vi "Teleop.vi"(10 "Match Info":T2={"Autonomous Elapsed Seconds"=0.0, "TeleOp Elapsed Seconds"=0.0, "Disabled Elapsed Seconds"=0.0, "Visited Autonomous"=FALSE, "Visited TeleOp"=FALSE, "Visited Disabled"=FALSE, "Autonomous Settings"={"Autonomous Style"=enum."Independent", "VI Refnum"=refnum}}, 11 "Call Context":T3) -> ()   [LabVIEW 2020]
doc: "This VI is called for each TeleOp packet received from the DS where the robot is not disabled. It is often used to read from the joysticks and update I/O or to update setpoints for timed control loops. It should complete and return within 20 milliseconds or it may miss DS packets."
uses:
  <vilib>/Rock Robotics/WPI/DriverStation/WPI_DriverStationDerivedRobotMode.ctl
  <vilib>/Rock Robotics/WPI/DriverStation/WPI_DriverStationMatch Info.ctl
  <vilib>/Rock Robotics/WPI/ThirdParty/Phoenix-LabVIEW/Motor Controller/Controls/CTRE_Phoenix_MotorControl_ControlMode.ctl
  <vilib>/Rock Robotics/WPI/Solenoid/WPI_SolenoidValue.ctl
  <vilib>/Rock Robotics/WPI/Utilities/WPI_GetSetVariantRefNum.vi
  <vilib>/Rock Robotics/Network Tables/NT Read Boolean.vi
  <vilib>/Rock Robotics/Network Tables/NT Read Number.vi
  <vilib>/Rock Robotics/WPI/Solenoid/WPI_SolenoidSetEnum.vi
  <vilib>/Rock Robotics/WPI/ThirdParty/Phoenix-LabVIEW/Motor Controller/Get/CTRE_Phoenix_MotorController_IntegratedSensorData_TalonFX.vi
  <vilib>/addons/control/pid/pid.llb/PID (DBL).vi
  <vilib>/Rock Robotics/Network Tables/NT Write Number.vi
  <vilib>/addons/control/pid/NI_PID_pid.lvlib
panel:
  in  "PID gains 5":T1={"proportional gain (Kc)"=0.005, "integral time (Ti, min)"=0.0, "derivative time (Td, min)"=2e-05} {"derivative time (Td, min)" format="%.6f"; "integral time (Ti, min)" format="%.3f"; "proportional gain (Kc)" format="%.3f"}
  in  "Subtract rpm":dbl=2975.0
  out "% voltage":dbl
  out "voltage (V)":dbl
  out "Motor Volts":dbl
  out "rpm":dbl
  out "limelight tx":dbl
  out "limelight ty":dbl
  in  "Auto-Accept":bool
  in  "8togglePressed?":bool
  out "Sample Slider 0":dbl(slide) scale=0.0..5.0
  out "Sample Boolean 1":bool
  out "Sample Boolean 0":bool
  # "-1"
  # "0"
  # ".75"
  # ".75"
  # "-.6"
  # "-.35"
  # ".1"
  # "1"
  # "-.1"
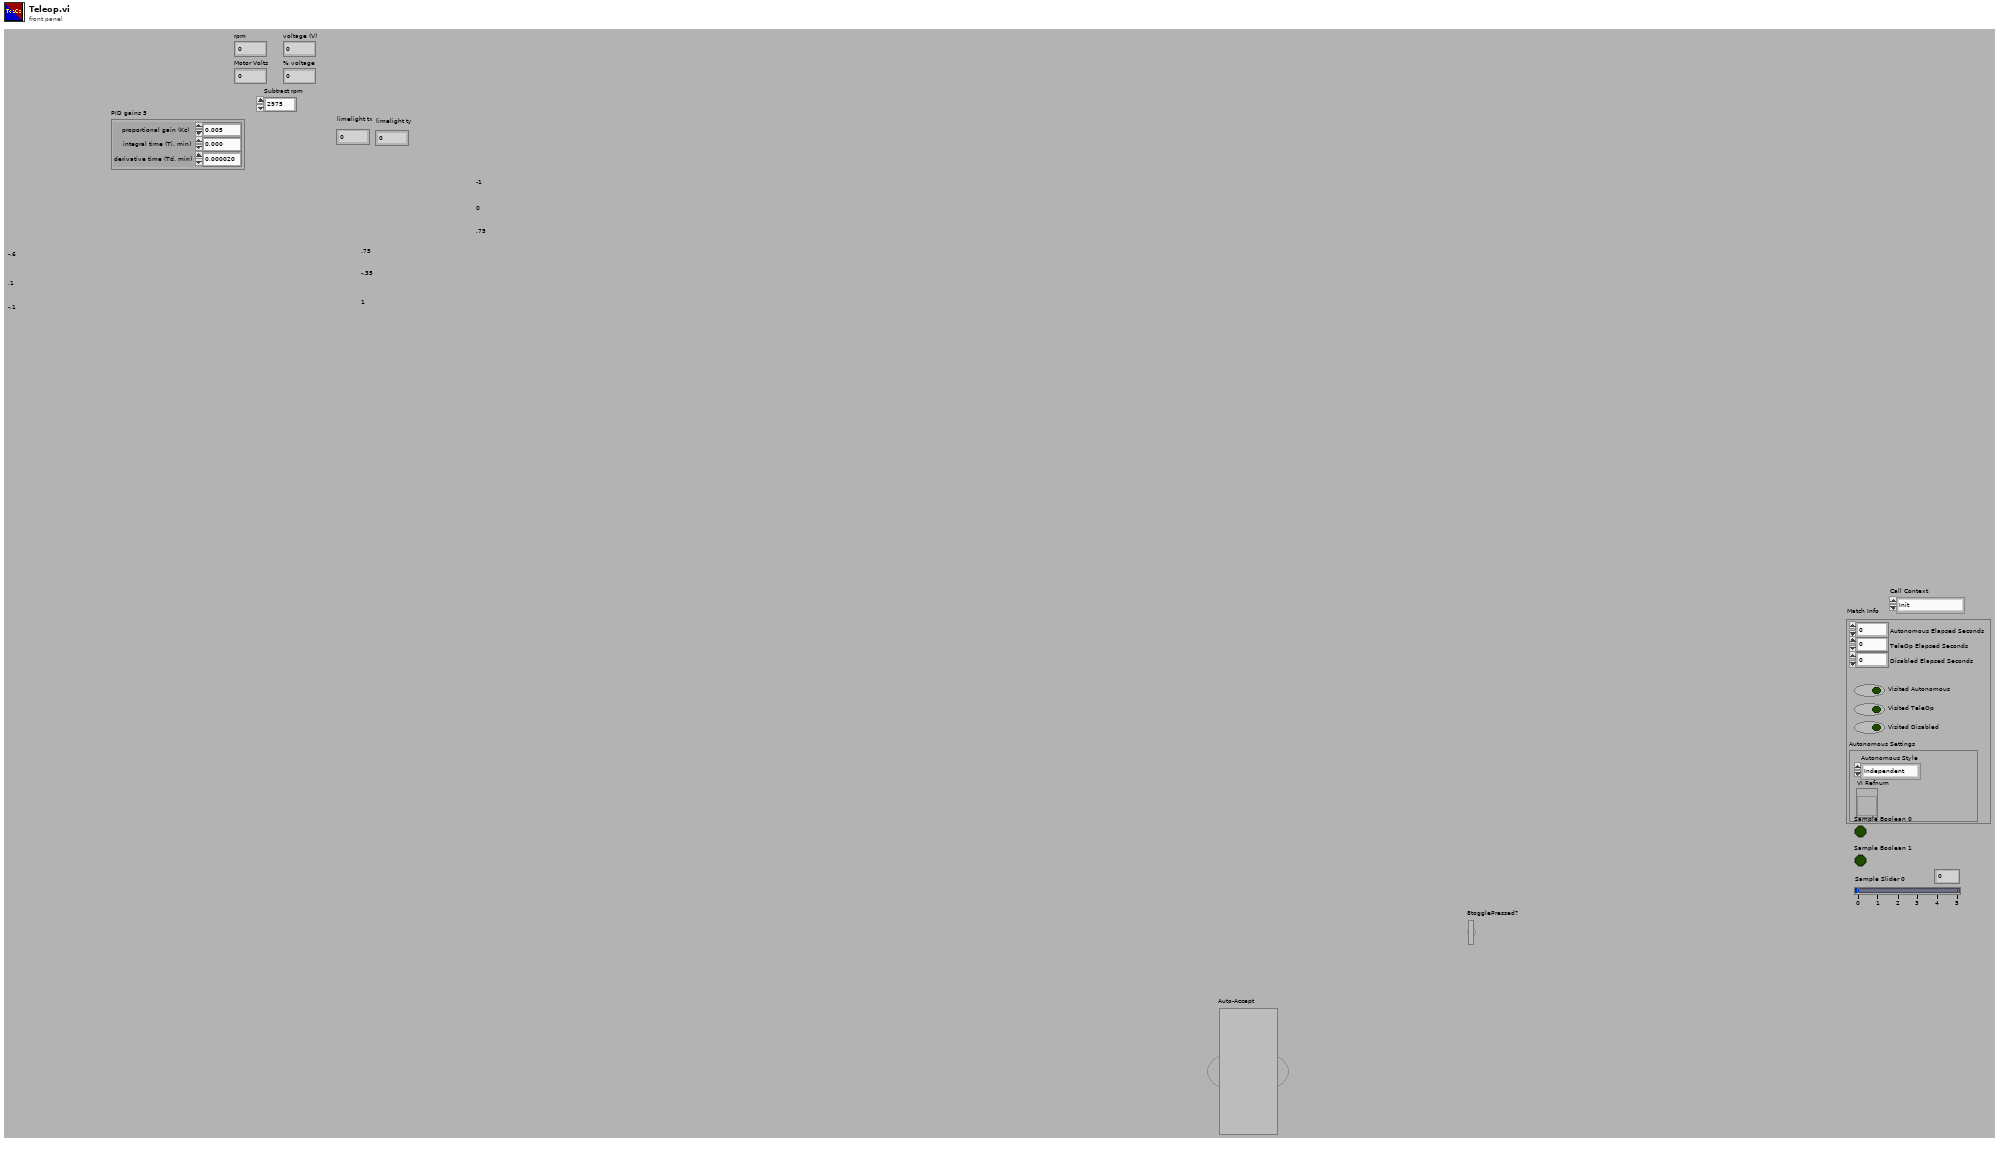
[diagram p1: front panel]
types:
  T1 = cluster{"proportional gain (Kc)":dbl, "integral time (Ti, min)":dbl, "derivative time (Td, min)":dbl}
  T2 = typedef "WPI_DriverStationMatch Info.ctl" = cluster{"Autonomous Elapsed Seconds":dbl, "TeleOp Elapsed Seconds":dbl, "Disabled Elapsed Seconds":dbl, "Visited Autonomous":bool, "Visited TeleOp":bool, "Visited Disabled":bool, "Autonomous Settings":cluster{"Autonomous Style":enum16{"Iterative", "Independent"}, "VI Refnum":refnum<vi>}}
  T3 = typedef "WPI_DriverStationDerivedRobotMode.ctl" = enum16{"Init", "Execute", "Stop"}
  T4 = typedef "CTRE_Phoenix_MotorControl_ControlMode.ctl" = u16
  T5 = typedef "WPI_SolenoidValue.ctl" = enum16{"Off", "On", "Forward", "Reverse"}
  T6 = typedef "WPI_MotorControlDeviceRef.ctl" = cluster{"DeviceStatus":errorcluster, "Type":T7, "PWM":cluster{"PWM Channel":T8, "DeadBand":T9}, "CAN":cluster{"Device Number":u8, "SetOutput VI Ref":variant, "GetOutput VI Ref":variant, "Enable VI Ref":variant, "Disable VI Ref":variant, "Data":variant}, "Invert":bool, "DIO PWM":cluster{"PWM \"Enable\" Channel":T8, "DIOChannel":T10, "PWM Rate":dbl}}
  T7 = typedef "WPI_MotorControlType.ctl" = enum16{"PWM", "CAN", "DIO PWM"}
  T8 = typedef "FPGA_DIOPWMChannel.ctl" = enum8{"PWM 0", "PWM 1", "PWM 2", "PWM 3", "PWM 4", "PWM 5", "PWM 6", "PWM 7", "PWM 8", "PWM 9", "PWM MXP 0", "PWM MXP 1", "PWM MXP 2", "PWM MXP 3", "PWM MXP 4", "PWM MXP 5", "PWM MXP 6", "PWM MXP 7", "PWM MXP 8", "PWM MXP 9", "Invalid"}
  T9 = typedef "WPI_PWMDeadband.ctl" = cluster{"Name":string, "maxPositivePwm":i32, "minPositivePwm":i32, "centerPwm":i32, "maxNegativePwm":i32, "minNegativePwm":i32, "angularRange":u16}
  T10 = typedef "FPGA_DIOChannel.ctl" = enum8{"DIO 0", "DIO 1", "DIO 2", "DIO 3", "DIO 4", "DIO 5", "DIO 6", "DIO 7", "DIO 8", "DIO 9", "DIO MXP 0", "DIO MXP 1", "DIO MXP 2", "DIO MXP 3", "DIO MXP 4", "DIO MXP 5", "DIO MXP 6", "DIO MXP 7", "DIO MXP 8", "DIO MXP 9", "DIO MXP 10", "DIO MXP 11", "DIO MXP 12", "DIO MXP 13", "DIO MXP 14", "DIO MXP 15", "SPI Port CS1", "SPI Port CS2", "SPI Port CS3", "SPI Port MISO", "SPI Port MOSI", "Invalid"}
  T11 = typedef "WPI_SolenoidDevRef.ctl" = cluster{"DevStatus":errorcluster, "Pneumatics Control Module":u8, "Forward Solenoid Channel":T12, "Reverse Solenoid Channel":T12}
  T12 = typedef "WPI_SolenoidChannel.ctl" = enum8{"Solenoid 0", "Solenoid 1", "Solenoid 2", "Solenoid 3", "Solenoid 4", "Solenoid 5", "Solenoid 6", "Solenoid 7", "Solenoid 8", "Solenoid 9", "Solenoid 10", "Solenoid 11", "Solenoid 12", "Solenoid 13", "Solenoid 14", "Solenoid 15", "Invalid"}
  T13 = typedef "WPI_CompressorDevRef.ctl" = cluster{"DevStatus":errorcluster, "Pneumatics Control Module":u8}
  T14 = typedef "WPI_SwitchDevRef.ctl" = cluster{"DevStatus":errorcluster, "DIO Channel":T10, "CntIndex":T15, "Normally Closed":bool}
  T15 = typedef "FPGA_CounterCtrSystemIndex.ctl" = enum8{"Ctr 0", "Ctr 1", "Ctr 2", "Ctr 3", "Ctr 4", "Ctr 5", "Ctr 6", "Ctr 7", "Invalid"}
  T16 = typedef "WPI_JoystickDevRef.ctl" = cluster{"Device":T17}
  T17 = typedef "WPI_JoystickDeviceEnum.ctl" = enum16{"USB 0", "USB 1", "USB 2", "USB 3", "USB 4", "USB 5"}
  T18 = cluster{"A":bool, "B":bool, "X":bool, "Y":bool, "Left Bumper":bool, "Right Bumper":bool, "View Button":bool, "Menu Button":bool, "Left Joystick Press":bool, "Right Joystick Press":bool, "Left Thumbpad X Axis":dbl, "Left Thumbpad Y Axis":dbl, "Left Trigger":dbl, "Right Trigger":dbl, "Right Thumbpad X Axis":dbl, "Right Thumbpad Y Axis":dbl, "Driver - Trigger":bool, "Driver - Middle Thumb":bool, "Driver - Left Thumb":bool, "Driver - Right Thumb":bool, "Driver - Left Top Left ":bool, "Driver - Left Top Middle":bool, "Driver - Left Top Right":bool, "Driver - Left Bottom Right":bool, "Driver - Left Bottom Middle":bool, "Driver - Left Bottom Left":bool, "Driver - Right Top Right":bool, "Driver - Right Top Middle":bool, "Driver - Right Top Left":bool, "Driver - Right Bottom Left":bool, "Driver - Right Bottom Middle":bool, "Driver - Right Bottom Right":bool, "Driver - X Axis":dbl, "Driver - Y Axis":dbl, "Driver - Z Axis":dbl}
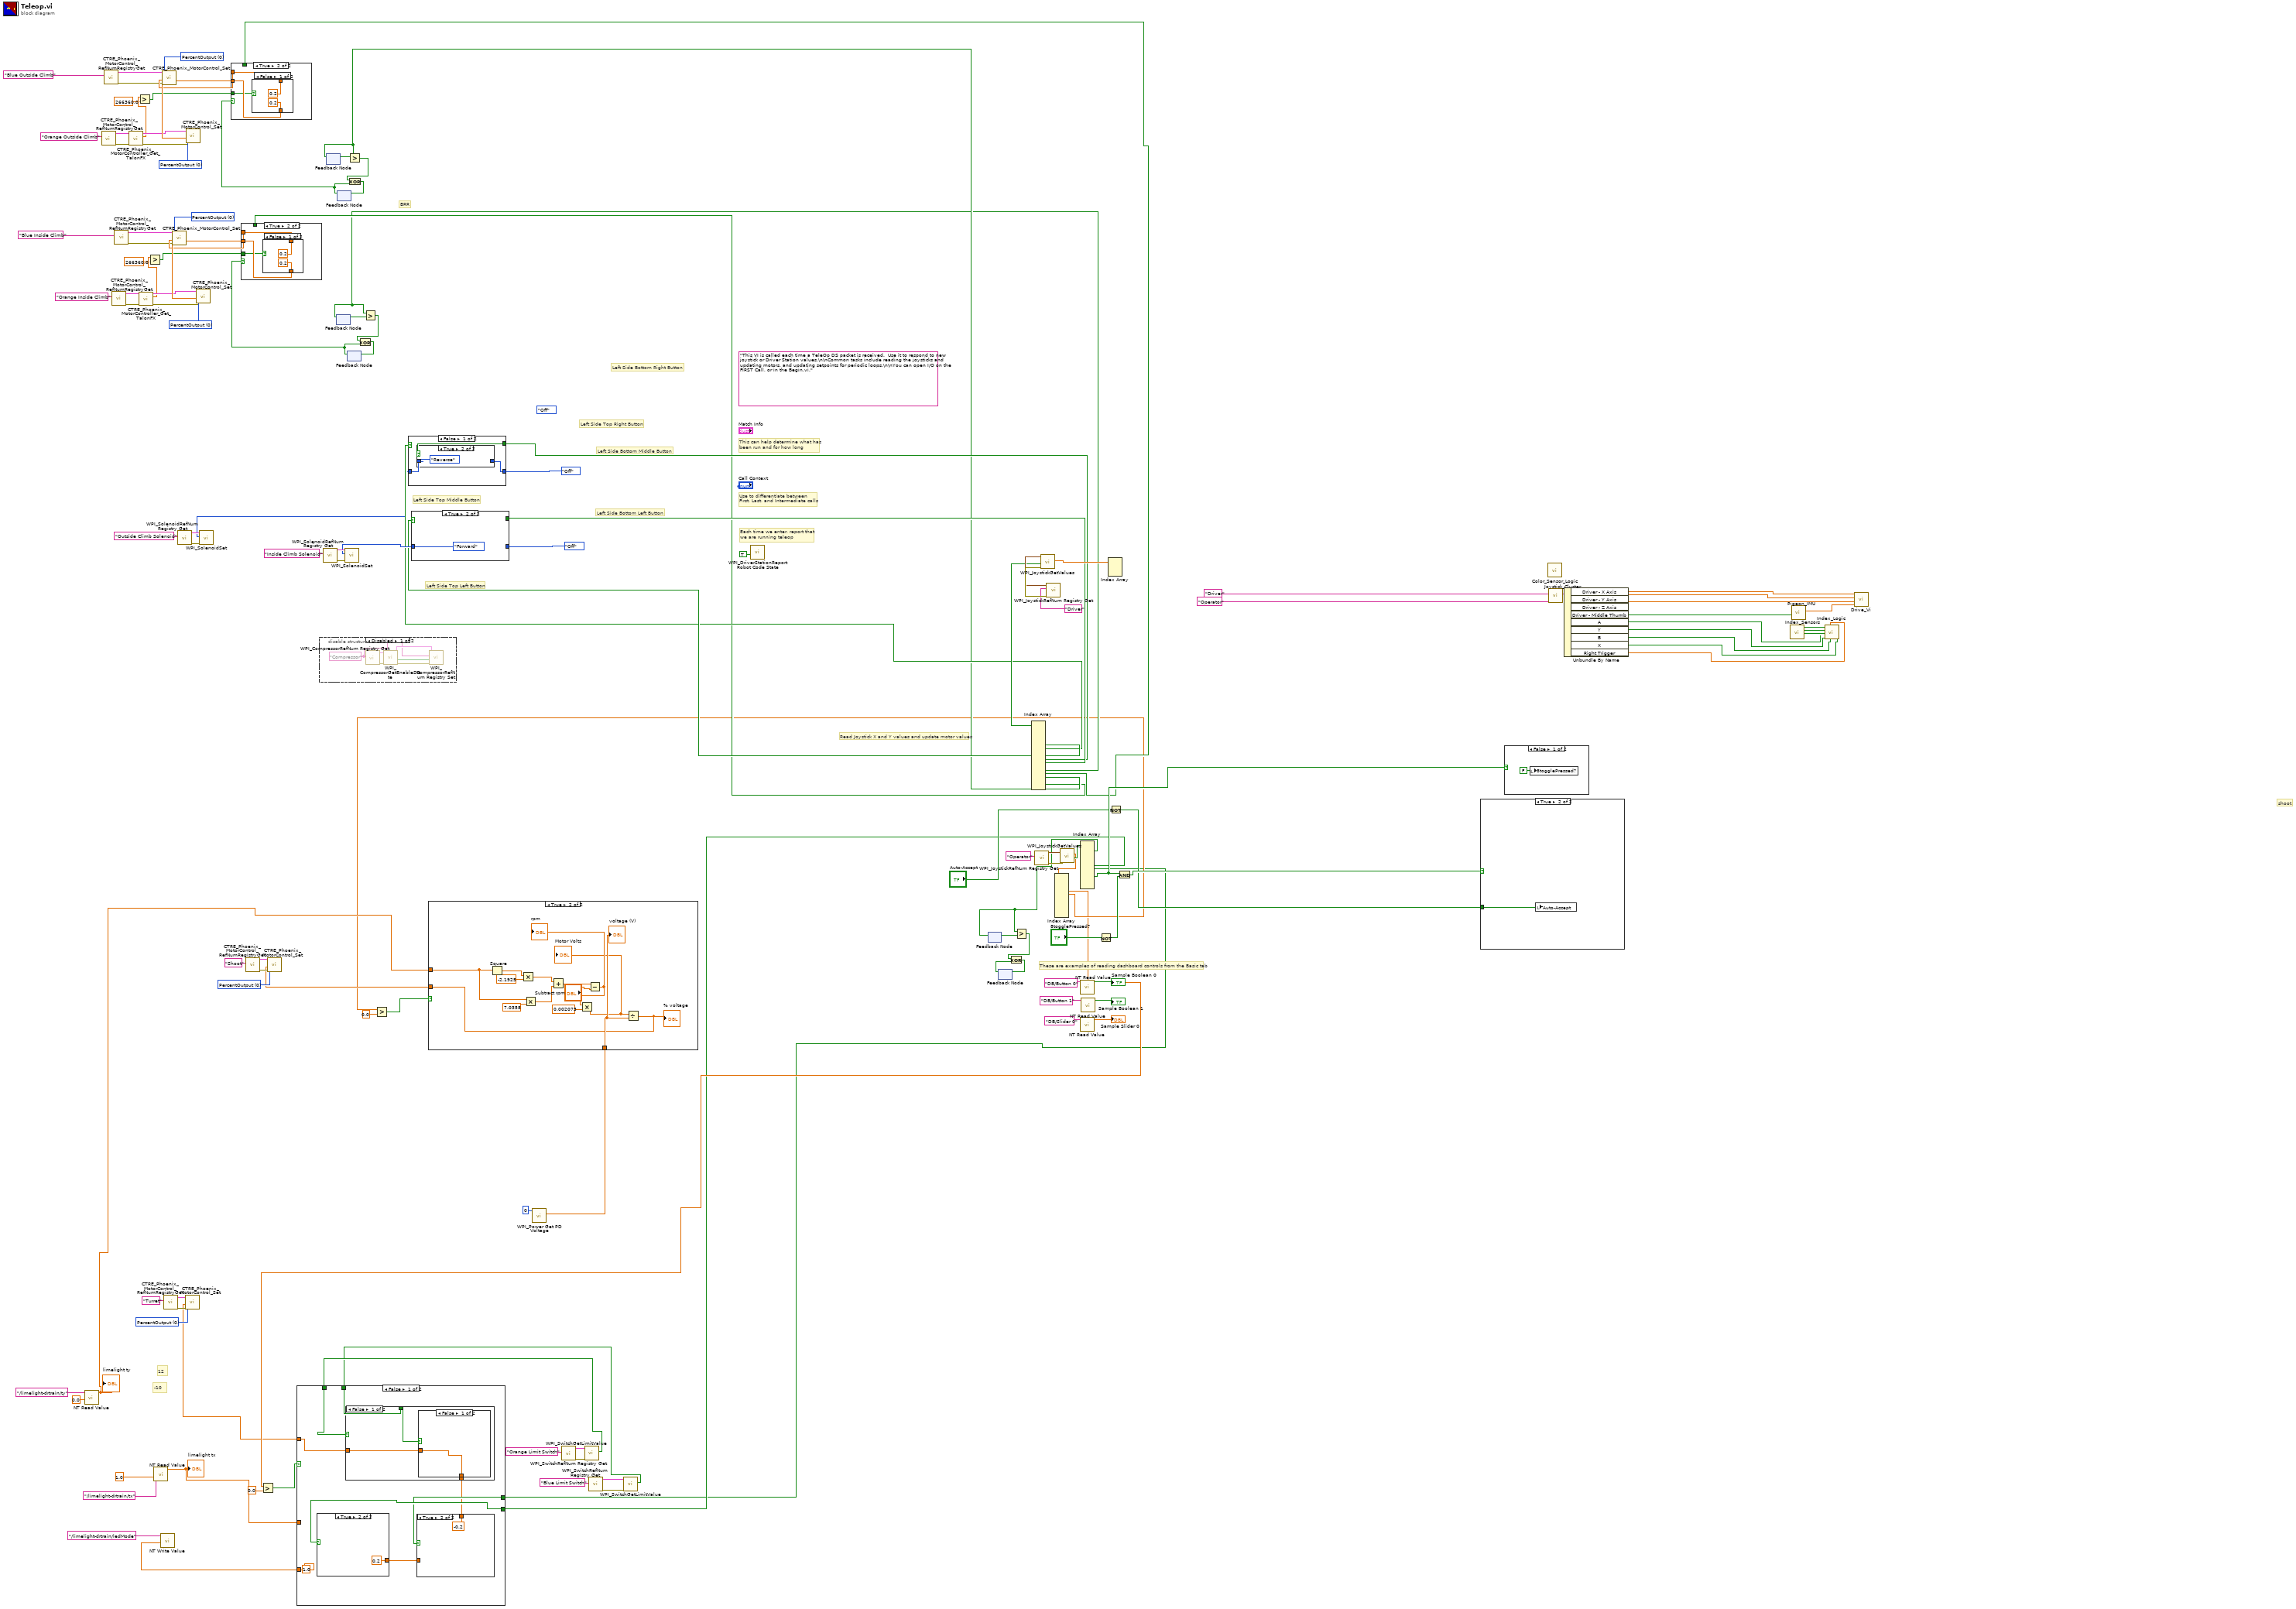
[diagram p0: block diagram]
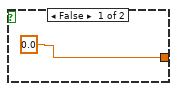
[diagram p3: hidden frame]
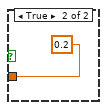
[diagram p4: hidden frame]
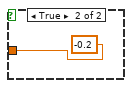
[diagram p5: hidden frame]
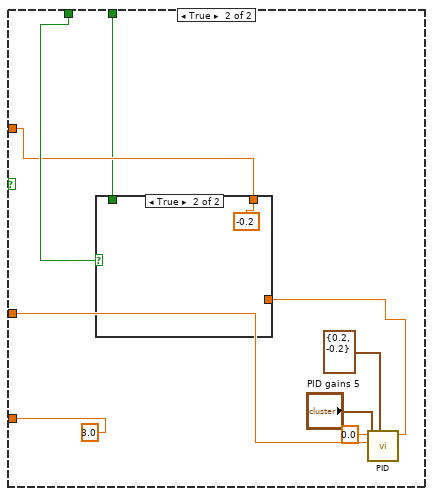
[diagram p6: hidden frame]
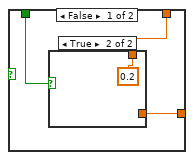
[diagram p7: hidden frame]
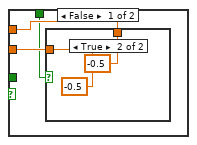
[diagram p9: hidden frame]
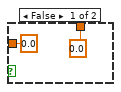
[diagram p10: hidden frame]
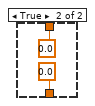
[diagram p11: hidden frame]
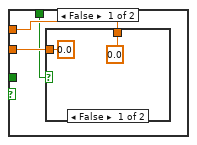
[diagram p12: hidden frame]
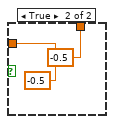
[diagram p13: hidden frame]
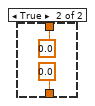
[diagram p14: hidden frame]
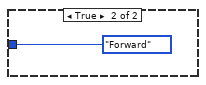
[diagram p17: hidden frame]
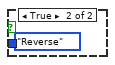
[diagram p19: hidden frame]
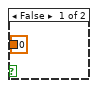
[diagram p20: hidden frame]
diagram:
  w52 = T4 0 items=["PercentOutput"=0, "Position"=1, "Velocity"=2, "Current"=3, "Follower"=5, "MotionProfile"=6, "MotionMagic"=7, "MotionProfileArc"=10, "Disabled"=15] ("Control Mode")
  w53 = T4 0 items=["PercentOutput"=0, "Position"=1, "Velocity"=2, "Current"=3, "Follower"=5, "MotionProfile"=6, "MotionMagic"=7, "MotionProfileArc"=10, "Disabled"=15] ("Control Mode")
  (unwired) WPI_SolenoidValue."Off" ("inside climb start")
  w71 = T4 0 items=["PercentOutput"=0, "Position"=1, "Velocity"=2, "Current"=3, "Follower"=5, "MotionProfile"=6, "MotionMagic"=7, "MotionProfileArc"=10, "Disabled"=15] ("Control Mode")
  w72 = T4 0 items=["PercentOutput"=0, "Position"=1, "Velocity"=2, "Current"=3, "Follower"=5, "MotionProfile"=6, "MotionMagic"=7, "MotionProfileArc"=10, "Disabled"=15] ("Control Mode")
  w102 = T4 0 items=["PercentOutput"=0, "Position"=1, "Velocity"=2, "Current"=3, "Follower"=5, "MotionProfile"=6, "MotionMagic"=7, "MotionProfileArc"=10, "Disabled"=15] ("Control Mode")
  w107 = T4 0 items=["PercentOutput"=0, "Position"=1, "Velocity"=2, "Current"=3, "Follower"=5, "MotionProfile"=6, "MotionMagic"=7, "MotionProfileArc"=10, "Disabled"=15] ("Control Mode")
  (unwired) "This VI is called each time a TeleOp DS packet is received.  Use it to respond to new joystick or Driver Station values.\n\nCommon tasks include reading the joysticks and updating motors, and updating setpoints for periodic loops.\n\nYou can open I/O on the FIRST Call, or in the Begin.vi."
  # "BRR"
  # "Left Side Bottom Right Button"
  # "Left Side Top Right Button"
  # "Left Side Bottom Middle Button"
  # "Left Side Top Middle Button"
  # "Left Side Bottom Left Button"
  # "Left Side Top Left Button"
  # "shoot"
  # "12"
  # "-10"
  # "These are examples of reading dashboard controls from the Basic tab"
  # "Read Joystick X and Y values and update motor values"
  # "Each time we enter, report that\nwe are running teleop"
  # "Use to differentiate between\nFirst, Last, and Intermediate calls"
  # "This can help determine what has\nbeen run and for how long"
  n1 = call-poly <vilib>:"NT Read Value.vi"("Default Value"=0.0, "Name"="/limelight-drtrain/ty") -> ("Numeric"=w83:dbl)  [unwired: 8 in, 1 out]
  "limelight ty" <- w83
  n2 = call <vilib>:"CTRE_Phoenix_MotorControl_RefNumRegistryGet.vi"("refnum name"="Orange Outside Climb") -> ("error out"=w49:errorcluster, "PhoenixMotorControlDevRef"=w48:T6)  [unwired: 9 in]
  n3 = call <vilib>:"CTRE_Phoenix_MotorControl_RefNumRegistryGet.vi"("refnum name"="Blue Outside Climb") -> ("error out"=w44:errorcluster, "PhoenixMotorControlDevRef"=w45:T6)  [unwired: 9 in]
  n4 = call <vilib>:"CTRE_Phoenix_MotorControl_RefNumRegistryGet.vi"("refnum name"="Orange Inside Climb") -> ("error out"=w68:errorcluster, "PhoenixMotorControlDevRef"=w67:T6)  [unwired: 9 in]
  n5 = call <vilib>:"CTRE_Phoenix_MotorControl_RefNumRegistryGet.vi"("refnum name"="Blue Inside Climb") -> ("error out"=w63:errorcluster, "PhoenixMotorControlDevRef"=w64:T6)  [unwired: 9 in]
  n6 = call-poly <vilib>:"CTRE_Phoenix_MotorController_Get_TalonFX.vi"("PhoenixMotorControlDevRef"=w48, "error in"=w49) -> ("PhoenixMotorControlDevRef"=w47:T6, "Position"=w39:dbl, "error out"=w46:errorcluster)  [unwired: 9 in, 2 out]
  n7 = Greater?(x=w39, y=266360.0) -> (0:w37:bool)
  n8 = call-poly <vilib>:"CTRE_Phoenix_MotorController_Get_TalonFX.vi"("PhoenixMotorControlDevRef"=w67, "error in"=w68) -> ("PhoenixMotorControlDevRef"=w66:T6, "Position"=w58:dbl, "error out"=w65:errorcluster)  [unwired: 9 in, 2 out]
  n9 = Greater?(x=w58, y=266360.0) -> (0:w56:bool)
  n10 = call-poly <vilib>:"NT Read Value.vi"("Default Value"=1.0, "Name"="/limelight-drtrain/tx") -> ("Numeric"=w24:dbl)  [unwired: 8 in, 1 out]
  "limelight tx" <- w24
  n11 = call <vilib>:"CTRE_Phoenix_MotorControl_RefNumRegistryGet.vi"("refnum name"="Turret") -> ("error out"=w105:errorcluster, "PhoenixMotorControlDevRef"=w104:T6)  [unwired: 9 in]
  n12 = call <vilib>:"WPI_SolenoidRefNum Registry Get.vi"("refnum name"="Outside Climb Solenoid") -> ("error out"=w97:errorcluster, "SolenoidDevRef"=w96:T11)  [unwired: 9 in]
  n13 = call <vilib>:"CTRE_Phoenix_MotorControl_RefNumRegistryGet.vi"("refnum name"="Shoot") -> ("error out"=w110:errorcluster, "PhoenixMotorControlDevRef"=w109:T6)  [unwired: 9 in]
  n14 = disable-structure shown="Disabled" {
    frame Disabled {
      w137 = "Compressor" ("refnum name")
      n15 = call <vilib>:"WPI_CompressorRefNum Registry Get.vi"("refnum name"=w137) -> ("error out"=w142:errorcluster, "CompressorDevRef"=w141:T13)  [unwired: 9 in]
      n16 = call <vilib>:"WPI_CompressorGetEnableState.vi"("error in (no error)"=w142, "CompressorDevRef"=w141) -> ("error out"=w140:errorcluster, "Compressor Running"=w139:bool, "CompressorDevRef"=w138:T13)  [unwired: 3 in, 4 out]
      n17 = call <vilib>:"WPI_CompressorRefNum Registry Set.vi"("error in (no error)"=w140, "Test Mode Only"=w139, "refnum name"=w137, "CompressorDevRef"=w138) -> ()  [unwired: 6 in, 2 out]
    }
    frame Enabled {
    }
  }
  n18 = call <vilib>:"WPI_SolenoidRefNum Registry Get.vi"("refnum name"="Inside Climb Solenoid") -> ("error out"=w94:errorcluster, "SolenoidDevRef"=w93:T11)  [unwired: 9 in]
  n19 = feedback #1() -> (w43:bool)  [unwired: 1 in]
  n20 = feedback #2() -> (w62:bool)  [unwired: 1 in]
  n21 = feedback #3() -> (w40:bool)  [unwired: 1 in]
  n22 = feedback #4() -> (w59:bool)  [unwired: 1 in]
  n23 = call <vilib>:"WPI_Power Get PD Voltage.vi"("Power Distribution Panel (def)"=u8 0) -> ("voltage (V)"=w84:dbl)  [unwired: 13 in, 1 out]
  n24 = call <vilib>:"WPI_SwitchRefNum Registry Get.vi"("refnum name"="Orange Limit Switch") -> ("error out"=w91:errorcluster, "SwitchDevRef"=w90:T14)  [unwired: 9 in]
  n25 = call <vilib>:"WPI_SwitchGetLimitValue.vi"("error in (no error)"=w91, "SwitchDevRef"=w90) -> ("Switch Pressed"=w22:bool)  [unwired: 7 in, 2 out]
  n26 = call <vilib>:"WPI_SwitchRefNum Registry Get.vi"("refnum name"="Blue Limit Switch") -> ("error out"=w88:errorcluster, "SwitchDevRef"=w87:T14)  [unwired: 9 in]
  n27 = call <vilib>:"WPI_SwitchGetLimitValue.vi"("error in (no error)"=w88, "SwitchDevRef"=w87) -> ("Switch Pressed"=w21:bool)  [unwired: 7 in, 2 out]
  n28 = call <vilib>:"WPI_DriverStationReport Robot Code State.vi"("TeleOp"=TRUE ("Autonomous")) -> ()  [unwired: 10 in, 1 out]
  n29 = feedback #5() -> (w114:bool)  [unwired: 1 in]
  n30 = feedback #6() -> (w36:bool)  [unwired: 1 in]
  n31 = call <vilib>:"WPI_JoystickRefNum Registry Get.vi"("refnum name"="Operator") -> ("error out"=w123:errorcluster, "JoystickDevRef"=w122:T16)  [unwired: 9 in]
  n32 = call <vilib>:"WPI_JoystickRefNum Registry Get.vi"("refnum name"="Driver") -> ("error out"=w135:errorcluster, "JoystickDevRef"=w134:T16)  [unwired: 9 in]
  n33 = call <vilib>:"WPI_JoystickGetValues.vi"("error in (no error)"=w135, "JoystickDevRef"=w134) -> ("Buttons"=w131:bool[], "Axes"=w132:dbl[])  [unwired: 5 in, 3 out]
  n34 = Index Array(array=w131) -> (element #5=w79:bool, element #6=w77:bool, element #9=w76:bool, element #10=w80:bool, element #12=w32:bool, element #13=w35:bool, element #14=w34:bool, element #16=w33:bool)  [unwired: 17 in, 9 out]
  n35 = case shown="True" w40 {
    tunnel: [w144 w151] -> w51
    tunnel: [w145 w152] -> w50
    tunnel: w35 -> [w143 _]
    tunnel: w37 -> [_ w150]
    frame False {
      n36 = case shown="True" w143 {
        tunnel: [0.0 ("Output") -0.5 ("Output")] -> w145
        tunnel: [0.0 ("Output") -0.5 ("Output")] -> w144
        frame False {
        }
        frame True {
        }
      }
    }
    frame True {
      n37 = case shown="False" w150 {
        tunnel: [0.2 ("Output") 0.0 ("Output")] -> w152
        tunnel: [0.2 ("Output") 0.0 ("Output")] -> w151
        frame False {
        }
        frame True {
        }
      }
    }
  }
  n38 = call <vilib>:"CTRE_Phoenix_MotorControl_Set.vi"("error in (no error)"=w44, "Output"=w50, "Control Mode"=w53, "PhoenixMotorControlDevRef"=w45) -> ()  [unwired: 6 in, 2 out]
  n39 = call <vilib>:"CTRE_Phoenix_MotorControl_Set.vi"("error in (no error)"=w46, "Output"=w51, "Control Mode"=w52, "PhoenixMotorControlDevRef"=w47) -> ()  [unwired: 6 in, 2 out]
  n40 = case shown="True" w59 {
    tunnel: [w158 w165] -> w70
    tunnel: [w159 w166] -> w69
    tunnel: w33 -> [w157 _]
    tunnel: w56 -> [_ w164]
    frame False {
      n41 = case shown="False" w157 {
        tunnel: [0.0 ("Output") -0.5 ("Output")] -> w159
        tunnel: [0.0 ("Output") -0.5 ("Output")] -> w158
        frame False {
        }
        frame True {
        }
      }
    }
    frame True {
      n42 = case shown="False" w164 {
        tunnel: [0.2 ("Output") 0.0 ("Output")] -> w166
        tunnel: [0.2 ("Output") 0.0 ("Output")] -> w165
        frame False {
        }
        frame True {
        }
      }
    }
  }
  n43 = call <vilib>:"CTRE_Phoenix_MotorControl_Set.vi"("error in (no error)"=w63, "Output"=w69, "Control Mode"=w72, "PhoenixMotorControlDevRef"=w64) -> ()  [unwired: 6 in, 2 out]
  n44 = call <vilib>:"CTRE_Phoenix_MotorControl_Set.vi"("error in (no error)"=w65, "Output"=w70, "Control Mode"=w71, "PhoenixMotorControlDevRef"=w66) -> ()  [unwired: 6 in, 2 out]
  n45 = feedback-in #1(w34) -> ()
  n46 = feedback-in #2(w32) -> ()
  n47 = Greater?(x=w34, y=w43) -> (0:w42:bool)
  n48 = Exclusive Or(1:w40, 2:w42) -> (0:w41:bool)
  n49 = feedback-in #3(w41) -> ()
  n50 = Greater?(x=w32, y=w62) -> (0:w61:bool)
  n51 = Exclusive Or(1:w59, 2:w61) -> (0:w60:bool)
  n52 = feedback-in #4(w60) -> ()
  n53 = case shown="False" w77 {
    tunnel: [w171 WPI_SolenoidValue."Forward" ("inside climb start")] -> w75
    tunnel: WPI_SolenoidValue."Off" ("inside climb start") -> [w172 _]
    tunnel: w76 -> [w173 _]
    frame False {
      n54 = case shown="True" w173 {
        tunnel: w172 -> [w174 _]
        tunnel: [w174 WPI_SolenoidValue."Reverse" ("inside climb start")] -> w171
        frame False {
        }
        frame True {
        }
      }
    }
    frame True {
    }
  }
  n55 = call-poly <vilib>:"WPI_SolenoidSet.vi"("error in (no error)"=w97, "Value"=w75, "SolenoidDevRef"=w96) -> ()  [unwired: 7 in, 2 out]
  n56 = case shown="True" w79 {
    tunnel: [w177 WPI_SolenoidValue."Forward" ("inside climb start")] -> w82
    tunnel: WPI_SolenoidValue."Off" ("inside climb start") -> [w178 _]
    tunnel: w80 -> [w179 _]
    frame False {
      n57 = case shown="False" w179 {
        tunnel: w178 -> [w180 _]
        tunnel: [w180 WPI_SolenoidValue."Reverse" ("inside climb start")] -> w177
        frame False {
        }
        frame True {
        }
      }
    }
    frame True {
    }
  }
  n58 = call-poly <vilib>:"WPI_SolenoidSet.vi"("error in (no error)"=w94, "Value"=w82, "SolenoidDevRef"=w93) -> ()  [unwired: 7 in, 2 out]
  n59 = call <vilib>:"WPI_JoystickGetValues.vi"("error in (no error)"=w123, "JoystickDevRef"=w122) -> ("Buttons"=w121:bool[], "Axes"=w31:dbl[])  [unwired: 5 in, 3 out]
  n60 = Index Array(array=w31) -> (element #3=w25:dbl, element #4=w28:dbl)  [unwired: 10 in, 8 out]
  n61 = Greater?(x=w25, y=0.0) -> (0:w26:bool)
  n62 = Greater?(x=w28, y=0.0) -> (0:w29:bool)
  n63 = case shown="True" w29 {
    tunnel: [0.0 ("Shoot %") w185] -> w106
    tunnel: w83 -> [_ w193]
    tunnel: w84 -> [_ w187]
    frame False {
    }
    frame True {
      n64 = Square(x=w193) -> (x^2=w196:dbl)
      n65 = Multiply(x=w196, y=-2.1925) -> (x*y=w194:dbl)
      n66 = Multiply(x=w193, y=7.0358) -> (x*y=w191:dbl)
      n67 = Add(x=w194, y=w191) -> (x+y=w190:dbl)
      n68 = Subtract(x=w190, y="Subtract rpm") -> (x-y=w189:dbl)
      "rpm" <- w189
      n69 = Multiply(x=w189, y=0.002075) -> (x*y=w186:dbl)
      "Motor Volts" <- w186
      n70 = Divide(x=w186, y=w187) -> (x/y=w185:dbl)
      "% voltage" <- w185
      "voltage (V)" <- w187
    }
  }
  n71 = call <vilib>:"CTRE_Phoenix_MotorControl_Set.vi"("error in (no error)"=w110, "Output"=w106, "Control Mode"=w107, "PhoenixMotorControlDevRef"=w109) -> ()  [unwired: 6 in, 2 out]
  n72 = Index Array(array=w121) -> (element #1=w113:bool, element #5=w20:bool, element #6=w19:bool, element #8=w116:bool)  [unwired: 11 in, 7 out]
  n73 = case shown="False" w26 {
    tunnel: w24 -> [_ w223]
    tunnel: [w198 w218] -> w23
    tunnel: w22 -> [w204 w219]
    tunnel: w21 -> [w203 w216]
    tunnel: w20 -> [w202 _]
    tunnel: w19 -> [w201 _]
    tunnel: [1.0 ("Numeric") 3.0 ("Numeric")] -> w17
    frame False {
      n74 = case shown="True" w202 {
        tunnel: [0.0 ("output") 0.2 ("output")] -> w200
        frame False {
        }
        frame True {
        }
      }
      n75 = case shown="True" w201 {
        tunnel: w200 -> [w205 _]
        tunnel: [w205 -0.2 ("output")] -> w199
        frame False {
        }
        frame True {
        }
      }
      n76 = case shown="False" w204 {
        tunnel: w203 -> [w211 _]
        tunnel: w199 -> [w210 _]
        tunnel: [w209 -0.2 ("output")] -> w198
        frame False {
          n77 = case shown="False" w211 {
            tunnel: w210 -> [w212 _]
            tunnel: [w212 0.2 ("output")] -> w209
            frame False {
            }
            frame True {
            }
          }
        }
        frame True {
        }
      }
    }
    frame True {
      n78 = call-poly <vilib>:"PID.vi"("output range"=cluster{"output high":dbl, "output low":dbl} {"output high"=0.2, "output low"=-0.2}, "PID gains"="PID gains 5", "process variable"=w223, "setpoint"=0.0) -> ("output"=w217:dbl)  [unwired: 6 in, 1 out]
      n79 = case shown="True" w219 {
        tunnel: [w225 -0.2 ("output")] -> w218
        tunnel: w217 -> [w224 _]
        tunnel: w216 -> [w226 _]
        frame False {
          n80 = case shown="True" w226 {
            tunnel: [w227 0.2 ("output")] -> w225
            tunnel: w224 -> [w227 _]
            frame False {
            }
            frame True {
            }
          }
        }
        frame True {
        }
      }
    }
  }
  n81 = call-poly <vilib>:"NT Write Value.vi"("Numeric"=w17, "Name"="/limelight-drtrain/ledMode") -> ()  [unwired: 9 in, 1 out]
  n82 = call <vilib>:"CTRE_Phoenix_MotorControl_Set.vi"("error in (no error)"=w105, "Output"=w23, "Control Mode"=w102, "PhoenixMotorControlDevRef"=w104) -> ()  [unwired: 6 in, 2 out]
  n83 = feedback-in #5(w113) -> ()
  n84 = Greater?(x=w113, y=w114) -> (0:w112:bool)
  n85 = Exclusive Or(1:w36, 2:w112) -> (0:w111:bool)
  n86 = feedback-in #6(w111) -> ()
  n87 = call-poly <vilib>:"NT Read Value.vi"("Name"="DB/Button 0" ("refnum name")) -> ("Boolean"=→"Sample Boolean 0":bool)  [unwired: 9 in, 1 out]
  n88 = call-poly <vilib>:"NT Read Value.vi"("Name"="DB/Slider 0" ("refnum name")) -> ("Numeric"=→"Sample Slider 0":dbl)  [unwired: 9 in, 1 out]
  n89 = call-poly <vilib>:"NT Read Value.vi"("Name"="DB/Button 1" ("refnum name")) -> ("Boolean"=→"Sample Boolean 1":bool)  [unwired: 9 in, 1 out]
  n90 = Not(x="8togglePressed?") -> (.not. x?=w119:bool)
  n91 = Index Array(array=w132) -> ()  [unwired: 3 in, 3 out]
  n92 = Not(x="Auto-Accept") -> (.not. x?=w117:bool)
  n93 = And(x=w116, y=w119) -> (x .and. y?=w118:bool)
  n94 = case shown="True" w118 {
    tunnel: w117 -> [_ w230]
    frame False {
    }
    frame True {
      n95 = local write "Auto-Accept"(w230) -> ()
    }
  }
  n96 = case shown="False" w116 {
    frame False {
      n97 = local write "8togglePressed?"(FALSE ("togglePressed?")) -> ()
    }
    frame True {
      n98 = local write "8togglePressed?"(TRUE ("togglePressed?")) -> ()
    }
  }
  n99 = call "Color_Sensor_Logic.vi"() -> ()  [unwired: 12 in]
  n100 = call "Joystick_Cluster.vi"("Xbox"="Operator", "Thrustmaster"="Driver") -> ("Joystick Output"=w14:T18)  [unwired: 9 in]
  n101 = Unbundle By Name(w14) -> ("Driver - X Axis"=w13:dbl, "Driver - Y Axis"=w12:dbl, "Driver - Z Axis"=w11:dbl, "Driver - Middle Thumb"=w10:bool, "A"=w5:bool, "Y"=w4:bool, "B"=w3:bool, "X"=w2:bool, "Right Trigger"=w1:dbl)
  n102 = call "Index_Sensors.vi"() -> ("Intake Pressed"=w8:bool, "Reject Pressed"=w7:bool, "Elevate Pressed"=w6:bool)  [unwired: 9 in]
  n103 = call "Pigeon_IMU.vi"("T/F"=w10) -> ("Yaw"=w9:dbl)  [unwired: 10 in]
  n104 = call "Index_Logic.vi"("X"=w2, "Intake Pressed"=w8, "B"=w3, "Right Trigger"=w1, "Y"=w4, "A"=w5, "Reject Pressed"=w7, "Elevate Pressed"=w6) -> ()  [unwired: 4 in]
  n105 = call "Drive_Vi.vi"("Yaw"=w9, "Z"=w11, "Y"=w12, "X"=w13) -> ()  [unwired: 8 in]
